vi "Hide_scanners.vi"(8 "error in":errorcluster, 9 "Y coordinate":dbl, 10 "X coordinate":dbl, 11 "task/channels in":refnum<k21>) -> (0 "error out":errorcluster, 3 "task out":refnum<k21>)   [LabVIEW 2021]
uses:
  <vilib>/Analysis/1siggen.llb/Ramp Pattern by Samples.vi
  <vilib>/DAQmx/write.llb/DAQmx Write (Analog 2D DBL NChan NSamp).vi
  <vilib>/DAQmx/configure/timing.llb/DAQmx Timing (Sample Clock).vi
  <vilib>/DAQmx/miscellaneous.llb/DAQmx Fill In Error Info.vi
  <vilib>/Analysis/NI_AALBase.lvlib
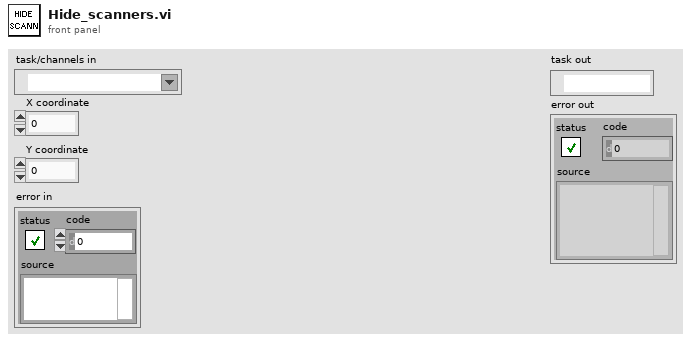
[diagram p1: front panel]
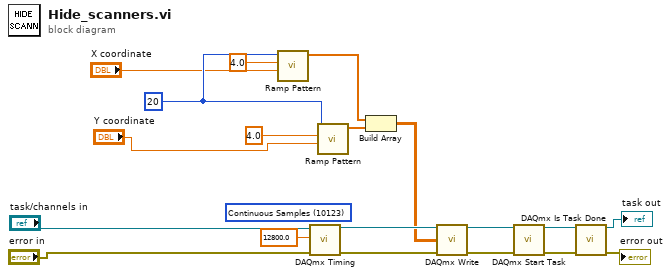
[diagram p0: block diagram]
diagram:
  w3 = 20 ("samples")
  (unwired) 10123 items=["Finite Samples"=10178, "Continuous Samples"=10123, "Hardware Timed Single Point"=12522] ("sample mode")
  n1 = call-poly <vilib>:"Ramp Pattern.vi"("start"="X coordinate", "end"=4.0, "samples"=w3) -> ("Ramp Pattern"=w6:dbl[])  [unwired: 7 in, 1 out]
  n2 = call-poly <vilib>:"DAQmx Timing.vi"("task/channels in"="task/channels in", "rate"=12800.0, "error in"="error in") -> ("task out"=w19:refnum<k21>, "error out"=w17:errorcluster)  [unwired: 11 in]
  n3 = call-poly <vilib>:"Ramp Pattern.vi"("start"="Y coordinate", "end"=4.0, "samples"=w3) -> ("Ramp Pattern"=w16:dbl[])  [unwired: 7 in, 1 out]
  n4 = Build Array(w6, w16) -> (w15:dbl[][])
  n5 = call-poly <vilib>:"DAQmx Write.vi"("task/channels in"=w19, "data"=w15, "error in"=w17) -> ("task out"=w14:refnum<k21>, "error out"=w13:errorcluster)  [unwired: 10 in, 1 out]
  n6 = call <vilib>:"DAQmx Start Task.vi"("task/channels in"=w14, "error in"=w13) -> ("task out"=w10:refnum<k21>, "error out"=w7:errorcluster)  [unwired: 12 in]
  n7 = call <vilib>:"DAQmx Is Task Done.vi"("task/channels in"=w10, "error in"=w7) -> ("task out"=→"task out":refnum<k21>, "error out"=→"error out":errorcluster)  [unwired: 11 in, 1 out]
